vi "measure_ratio_signal.vi"(8 "error in":errorcluster, 10 "Measurement settings":T1={"Start Wavelength (nm)"=300.0, "End Wavelength (nm)"=900.0, "Increment (nm)"=5.0, "White Bias (No. of Suns)"=1.0, "Averages per wavlength"=1.0, "Time Constant"=8, "Low Pass Filter Slope "=1, "Gain (V/A)"=50.0} {"Gain (V/A)" format="%#.2f"; "Low Pass Filter Slope" items=["6 dB/oct", "12 dB/oct", "18 db/oct", "24 dB/oct"]; "Time Constant" items=["10 us", "30 us", "100 us", "300 us", "1 ms", "3 ms", "10 ms", "30 ms", "100 ms", "300 ms", "1 s", "3 s", "10 s", "30 s", "100 s", "300 s", "1 ks", "3 ks", "10 ks", "30 ks"]; "Averages per wavlength" format="%#.2f"; "White Bias (No. of Suns)" format="%#.2f"; "End Wavelength (nm)" min=350.0 max=1100.0 format="%#.2f"; "Start Wavelength (nm)" min=350.0 max=1100.0 format="%#.2f"}, 11 "VISA resource name in":refnum<visa-resource-name>="GPIB0::8::INSTR") -> (0 "error out":errorcluster, 2 "Averaged scaled ratio":dbl, 3 "VISA resource name out":refnum<visa-resource-name>)   [LabVIEW 2018]
uses:
  typedefs/measurement_settings.ctl
  <instrlib>/Stanford Research 830/Public/Data/Read (1 Parameter).vi
  <instrlib>/Stanford Research 830/Stanford Research 830.lvlib
panel:
  out "Raw ratio":dbl
  out "Intensity-graph":T2(graph)
  out "Ratio (%)":dbl
  # "Wavelength average intensity"
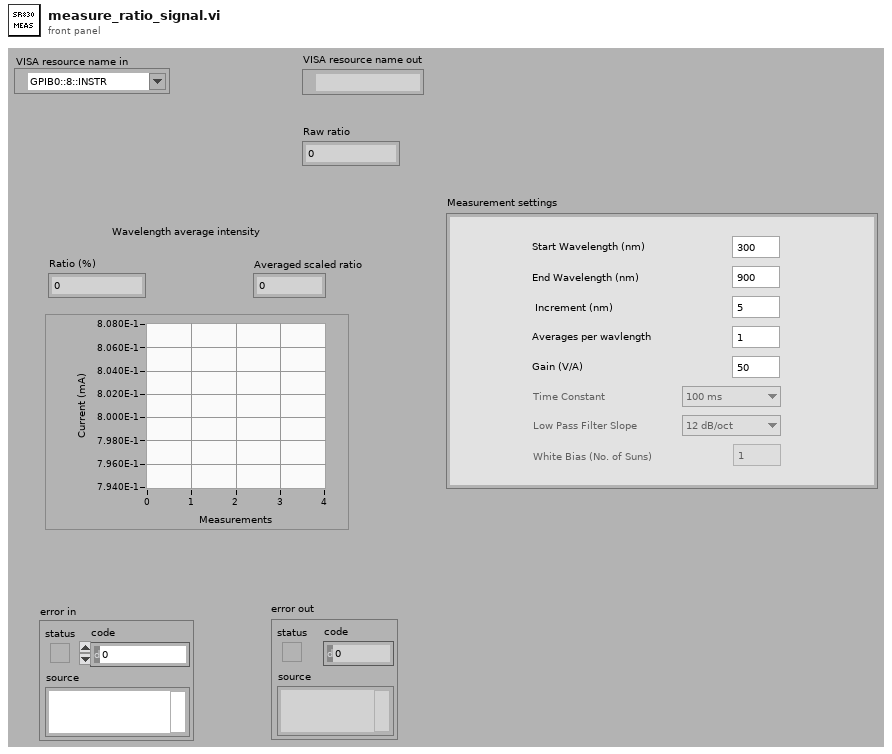
[diagram p1: front panel]
types:
  T1 = typedef "measurement_settings.ctl" = cluster{"Start Wavelength (nm)":dbl, "End Wavelength (nm)":dbl, "Increment (nm)":dbl, "White Bias (No. of Suns)":dbl, "Averages per wavlength":dbl, "Time Constant":u16, "Low Pass Filter Slope ":u16, "Gain (V/A)":dbl}
  T2 = cluster{"meas_index 2":i32[], "Intensity 3":dbl[]}
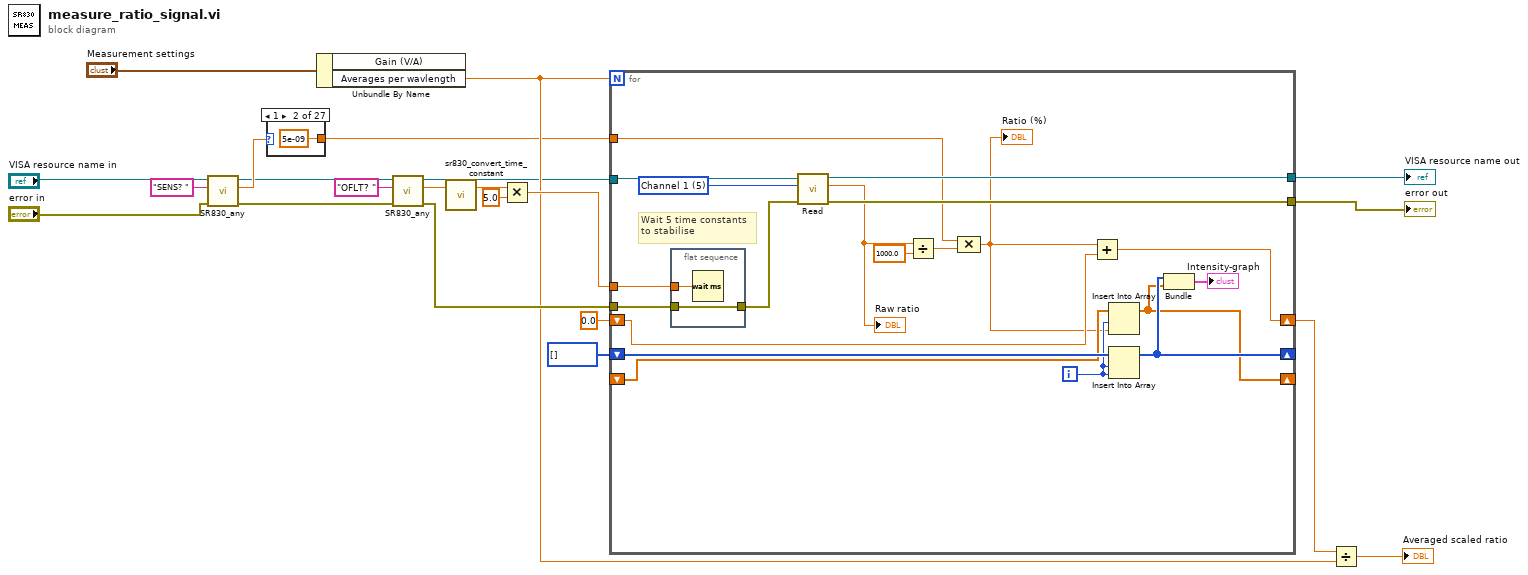
[diagram p0: block diagram]
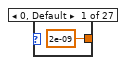
[diagram p2: hidden frame]
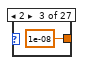
[diagram p3: hidden frame]
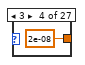
[diagram p4: hidden frame]
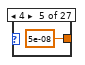
[diagram p5: hidden frame]
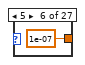
[diagram p6: hidden frame]
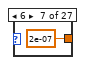
[diagram p7: hidden frame]
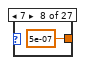
[diagram p8: hidden frame]
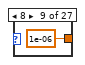
[diagram p9: hidden frame]
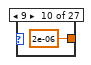
[diagram p10: hidden frame]
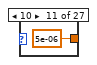
[diagram p11: hidden frame]
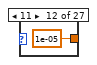
[diagram p12: hidden frame]
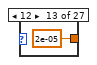
[diagram p13: hidden frame]
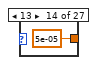
[diagram p14: hidden frame]
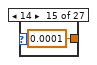
[diagram p15: hidden frame]
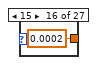
[diagram p16: hidden frame]
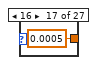
[diagram p17: hidden frame]
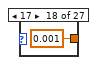
[diagram p18: hidden frame]
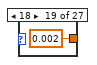
[diagram p19: hidden frame]
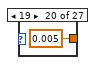
[diagram p20: hidden frame]
diagram:
  n1 = call "SR830_any.vi"("error in (no error)"="error in", "initial string"="SENS? ", "VISA resource name"="VISA resource name in") -> ("error out"=w4:errorcluster, "Measurement"=w6:dbl, "VISA resource name out"=w5:refnum<visa-resource-name>)  [unwired: 6 in]
  n2 = case shown="1" w6 {
    tunnel: [2e-09 5e-09 1e-08 2e-08 5e-08 1e-07 2e-07 5e-07 1e-06 2e-06 5e-06 1e-05 2e-05 5e-05 0.0001 0.0002 0.0005 0.001 0.002 0.005 0.01 0.02 0.05 0.1 0.2 0.5 1] -> w1
    frame 0, Default {
    }
    frame 1 {
    }
    frame 2 {
    }
    frame 3 {
    }
    frame 4 {
    }
    frame 5 {
    }
    frame 6 {
    }
    frame 7 {
    }
    frame 8 {
    }
    frame 9 {
    }
    frame 10 {
    }
    frame 11 {
    }
    frame 12 {
    }
    frame 13 {
    }
    frame 14 {
    }
    frame 15 {
    }
    frame 16 {
    }
    frame 17 {
    }
    frame 18 {
    }
    frame 19 {
    }
    frame 20 {
    }
    frame 21 {
    }
    frame 22 {
    }
    frame 23 {
    }
    frame 24 {
    }
    frame 25 {
    }
    frame 26 {
    }
  }
  n3 = Unbundle By Name("Measurement settings") -> ("Averages per wavlength"=w9:dbl)  [unwired: 1 out]
  n4 = call "SR830_any.vi"("error in (no error)"=w4, "initial string"="OFLT? ", "VISA resource name"=w5) -> ("error out"=w14:errorcluster, "Measurement"=w15:dbl, "VISA resource name out"=w8:refnum<visa-resource-name>)  [unwired: 6 in]
  n5 = call "sr830_convert_time_constant.vi"("Time constant code"=w15) -> ("time constant  in ms"=w19:dbl)  [unwired: 2 in]
  n6 = Multiply(x=w19, y=5.0) -> (x*y=w17:dbl)
  n7 = for {
    N: w9 -> [_]
    tunnel: w8 -> [w56]
    tunnel: [w55] -> w21
    tunnel: [w69] -> w20
    shift-right: [w63] -> w13
    shift-left: 0.0 -> [w60]
    shift-right: [w62] -> _
    shift-left: i32[] [] -> [w67]
    shift-right: [w61] -> _
    shift-left: _ -> [w66]
    tunnel: w17 -> [w59]
    tunnel: w14 -> [w58]
    tunnel: w1 -> [w54]
    i -> [w65]
    w68 = u16 5 items=["X"=1, "Y"=2, "R"=3, "Theta"=4, "Channel 1"=5, "Channel 2"=6, "Aux In 1"=7, "Aux In 2"=8, "Aux In 3"=9, "Aux In 4"=10] ("Parameter (1: X)")
    # "Wait 5 time constants\nto stabilise"
    n8 = flat-sequence {
      tunnel: w59 -> [w71]
      tunnel: w58 -> [w70]
      tunnel: [w70] -> w57
      frame #0 {
        n9 = Wait (ms)(milliseconds to wait=w71) -> ()  [unwired: 1 out]
      }
    }
    n10 = call-poly <instrlib>:"Read.vi"("error in (no error)"=w57, "Parameter (1: X)"=w68, "VISA resource name"=w56) -> ("error out"=w69:errorcluster, "Measurement"=w51:dbl, "VISA resource name out"=w55:refnum<visa-resource-name>)  [unwired: 6 in]
    "Raw ratio" <- w51
    n11 = Divide(x=w51, y=1000.0) -> (x/y=w52:dbl)
    n12 = Compound Arithmetic op=MULTIPLY(w54, w52) -> (w53:dbl)
    "Ratio (%)" <- w53
    n13 = Add(x=w53, y=w60) -> (x+y=w63:dbl)
    n14 = Insert Into Array(array=w66, index=w65, new element=w53) -> (w61:dbl[])
    n15 = Insert Into Array(array=w67, index=w65, new element=w65) -> (w62:i32[])
    n16 = Bundle(w62, w61) -> (→"Intensity-graph":cluster{i32[], dbl[]})  [unwired: 1 in]
  }
  "VISA resource name out" <- w21
  "error out" <- w20
  n17 = Divide(x=w13, y=w9) -> (x/y=→"Averaged scaled ratio":dbl)
